vi "DEV Write User Data.vi"(7 "DataLen":i32, 9 "pWriteData":u8[](array[numeric])=array[4097 elements], 10 "OffsetAddr":i32, 11 "DevHandle":i32) -> (1 "pWriteData out":u8[](array[numeric]), 3 "function return":bool)   [LabVIEW 2010, in "usb_device.lvlib"]
doc: "bool WINAPI DEV_WriteUserData(int DevHandle,int OffsetAddr,unsigned char *pWriteData,int DataLen);"
uses:
  usb_device.lvlib
  USB2XXX.dll
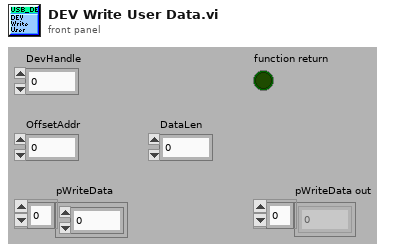
[diagram p1: front panel]
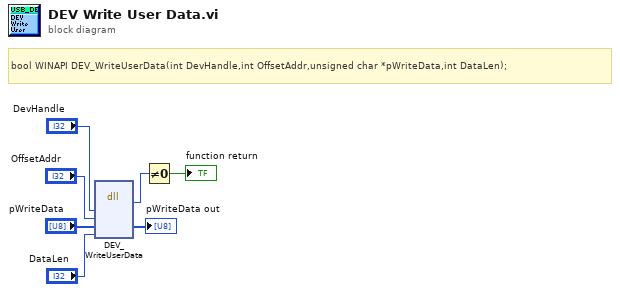
[diagram p0: block diagram]
diagram:
  # "bool WINAPI DEV_WriteUserData(int DevHandle,int OffsetAddr,unsigned char *pWriteData,int DataLen);"
  n1 = dll-call lib="G:/OtherWork/USB2XXX_Example/trunk/Labview/PublicFiles/USB2XXX.*" fn="DEV_WriteUserData"("DevHandle"="DevHandle", "OffsetAddr"="OffsetAddr", "pWriteData"="pWriteData", "DataLen"="DataLen") -> (w6:u8, "pWriteData"=→"pWriteData out":u8[])  [unwired: 6 in, 2 out]
  n2 = Not Equal To 0?(x=w6) -> (x != 0?=→"function return":bool)
